vi "HEWH 5 Second After Draw.vi"(6 "Seconds to Remove":T2, 7 "Remove from location":T1, 11 "Software Elapsed Time (s) in":dbl[](array[numeric]) format="%#.6f") -> (2 "Time (15 sec After)":dbl, 3 "Software Elapsed Time (s) out":dbl[](array[numeric]), 4 "Time Index":i32)   [LabVIEW 2023]
uses:
  Type Definitions/HEWH Seconds to Remove.ctl
  Type Definitions/HEWH Remove From Location.ctl
panel:
  out "Difference (Debug)":dbl
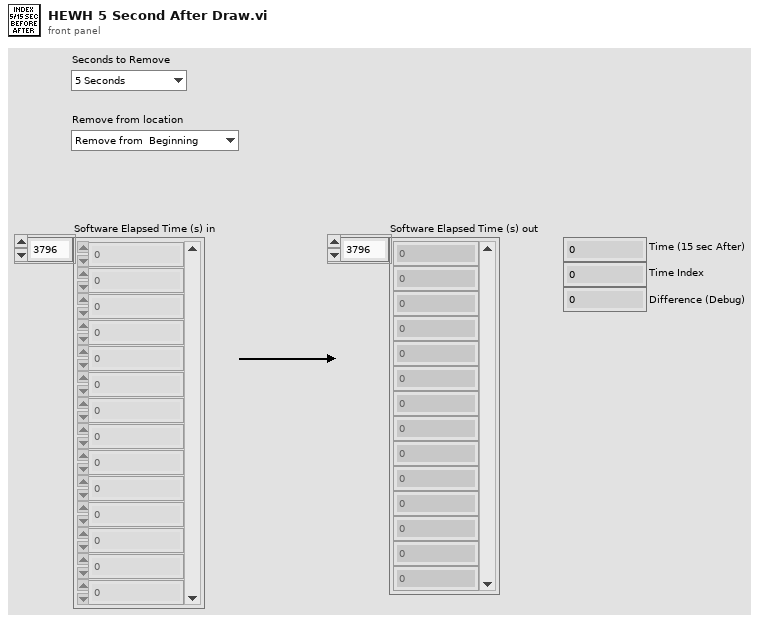
[diagram p1: front panel]
types:
  T1 = typedef "HEWH Remove From Location.ctl" = enum16{"Remove from  Beginning", "Remove from End"}
  T2 = typedef "HEWH Seconds to Remove.ctl" = enum16{"5 Seconds", "15 Seconds"}
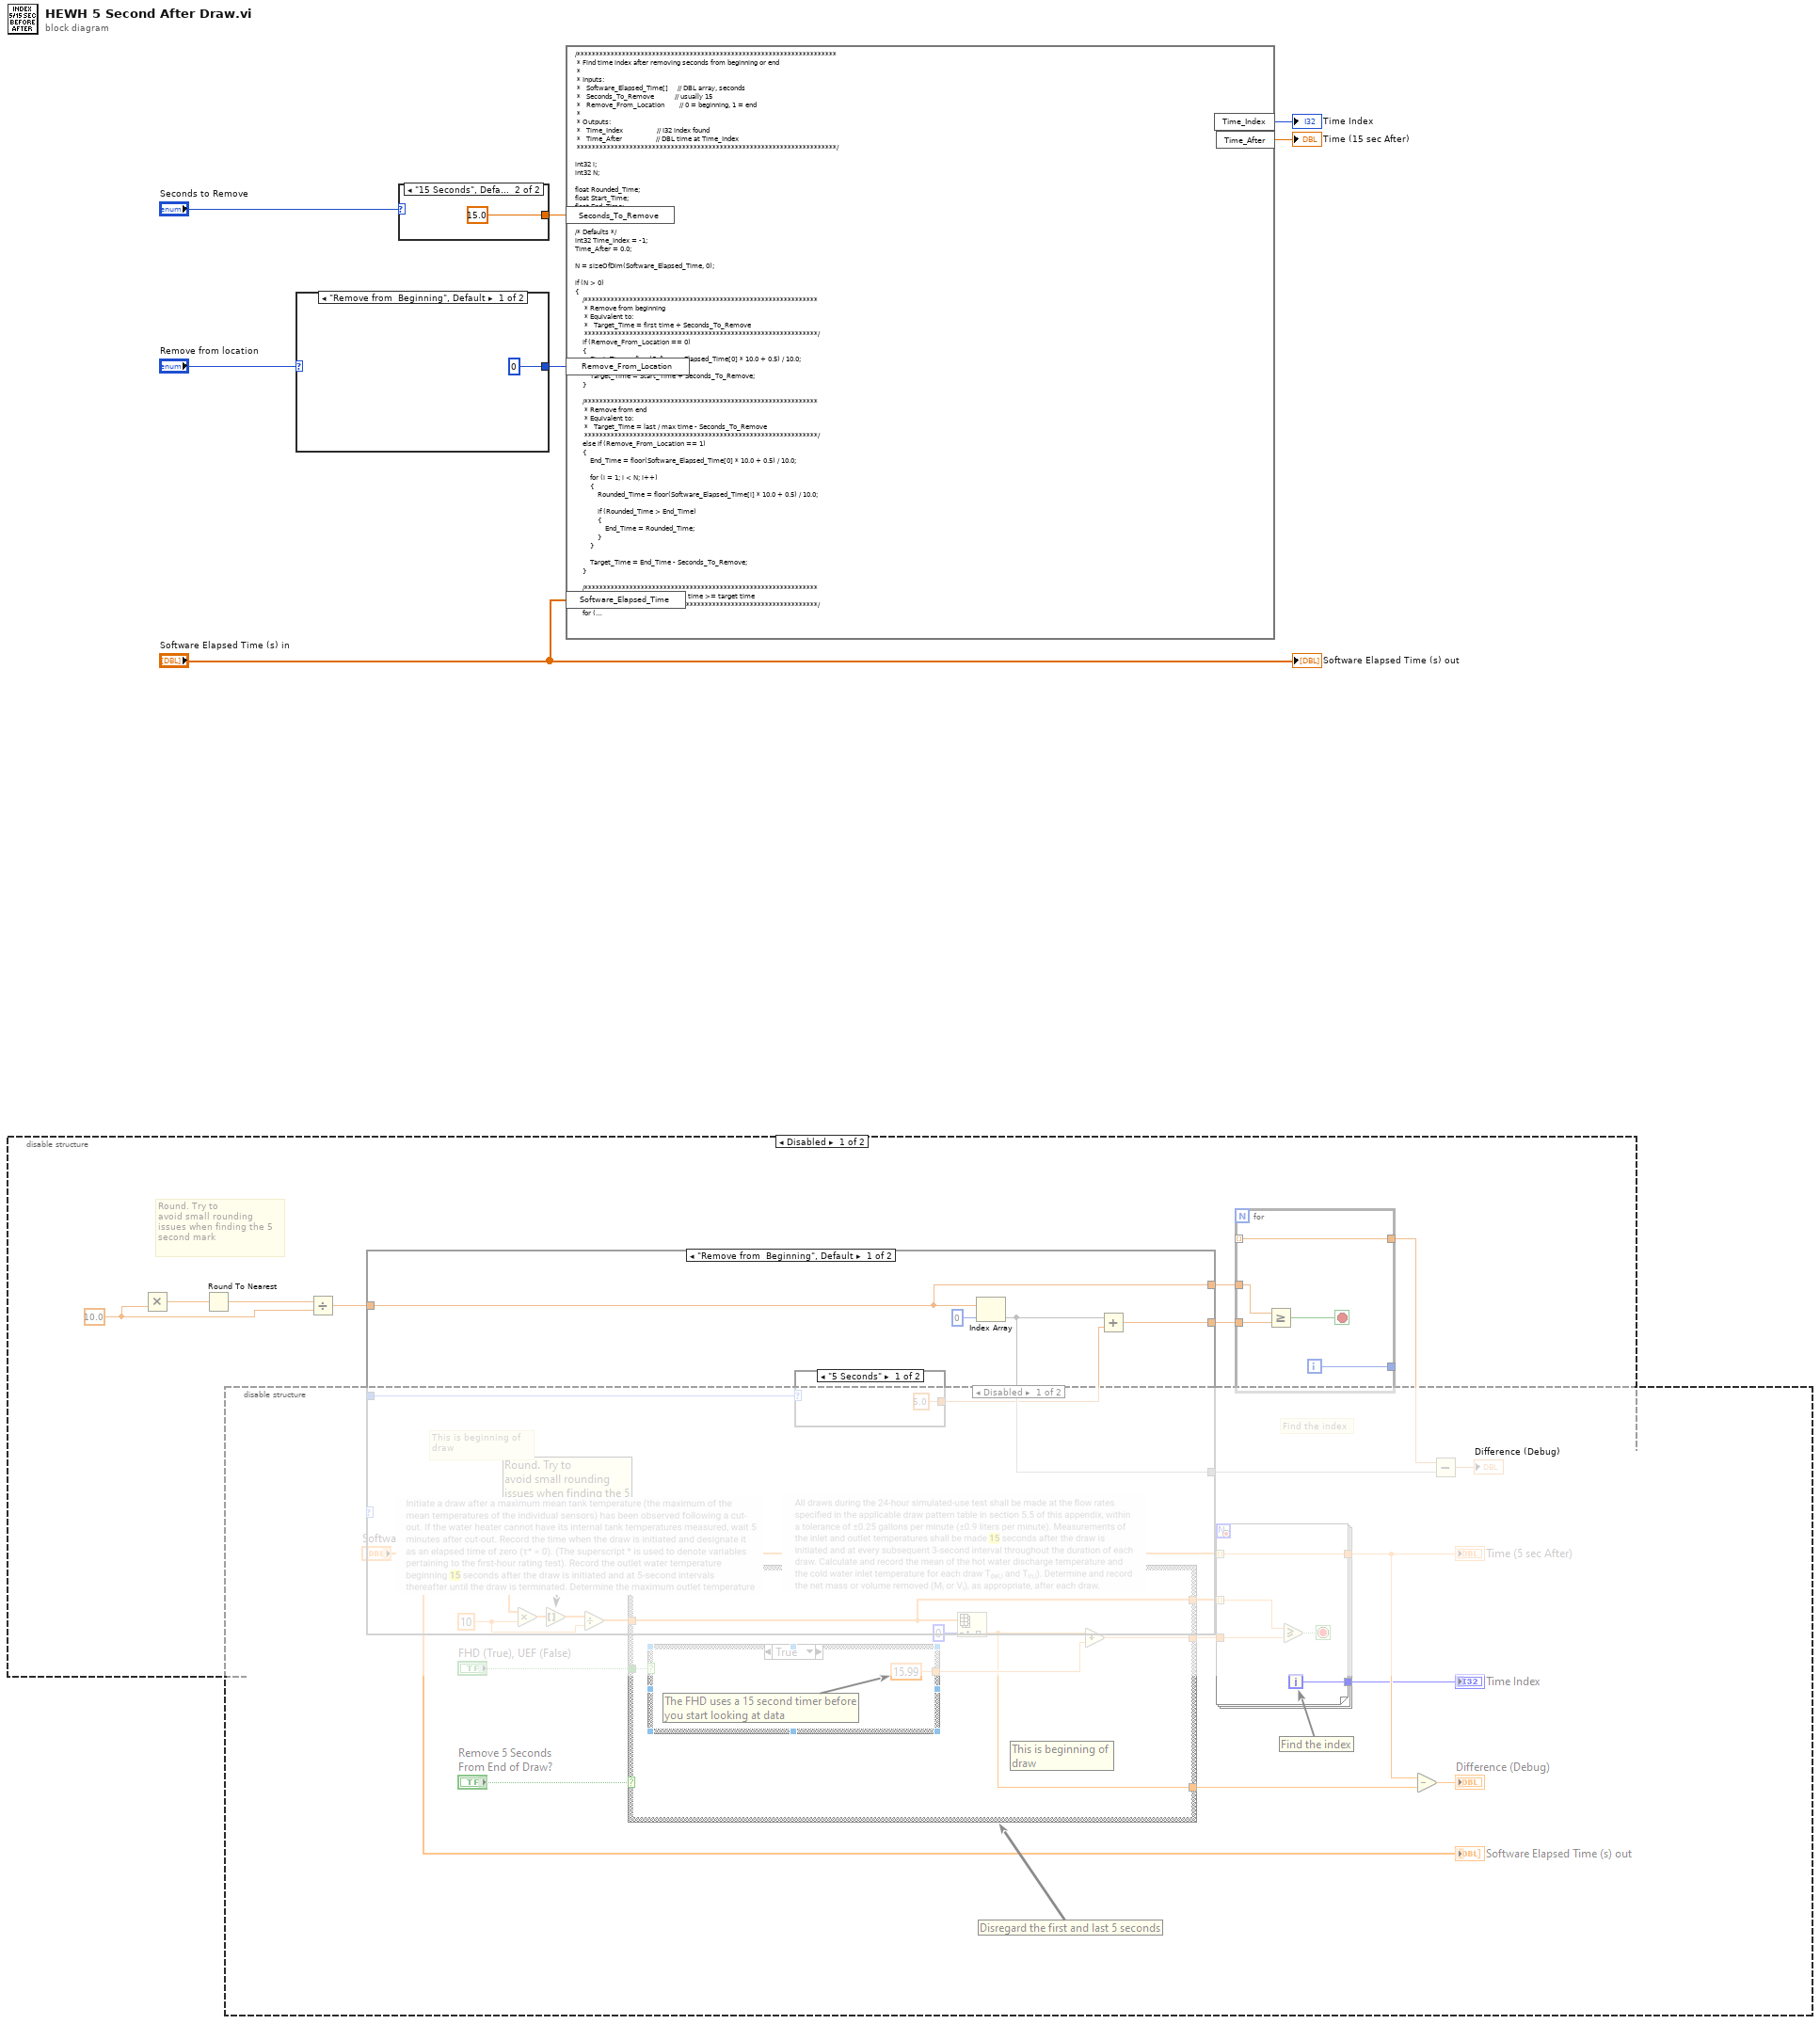
[diagram p0: block diagram]
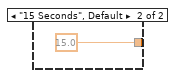
[diagram p2: hidden frame]
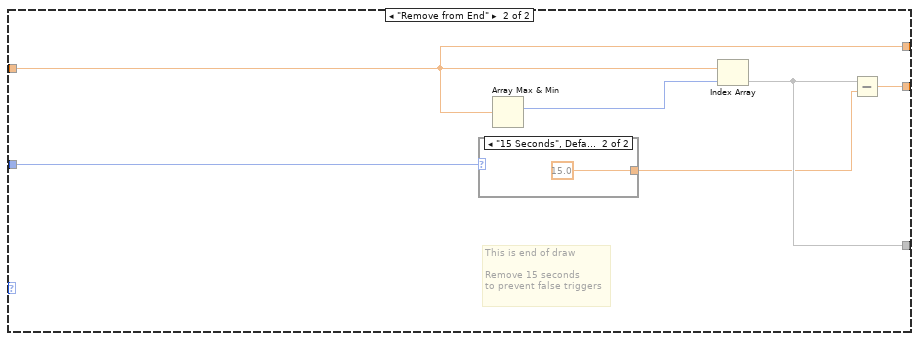
[diagram p3: hidden frame]
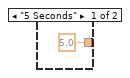
[diagram p4: hidden frame]
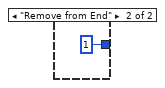
[diagram p6: hidden frame]
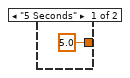
[diagram p7: hidden frame]
diagram:
  n1 = disable-structure shown="Disabled" {
    frame Disabled {
      w16 = 10.0
      # "Find the index"
      # "Round. Try to\navoid small rounding\nissues when finding the 5\nsecond mark"
      n2 = Multiply(y=w16) -> (x*y=w14:dbl)  [unwired: 1 in]
      n3 = Round To Nearest(number=w14) -> (nearest integer value=w15:dbl)
      n4 = Divide(x=w15, y=w16) -> (x/y=w12:dbl)
      n5 = case shown="\"Remove from  Beginning\", Default" {
        selector: _ -> [_ _]
        tunnel: [w22 w30] -> w13
        tunnel: w12 -> [w20 w29]
        tunnel: [w20 w29] -> w11
        tunnel: [w19 w27] -> w9
        tunnel: _ -> [w17 w26]
        frame "Remove from  Beginning", Default {
          # "This is beginning of \ndraw"
          n6 = case shown="\"5 Seconds\"" w17 {
            tunnel: [5.0 ("Ignore Seconds at Beginning") 15.0 ("Ignore Seconds at Beginning")] -> w18
            frame "5 Seconds" {
            }
            frame "15 Seconds", Default {
            }
          }
          n7 = Index Array "Index Array"(array=w20, index=0) -> (element=w19)
          n8 = Add(x=w19, y=w18) -> (x+y=w22:dbl)
        }
        frame "Remove from End" {
          # "This is end of draw\n\nRemove 15 seconds\nto prevent false triggers"
          n9 = case shown="\"15 Seconds\", Default" w26 {
            tunnel: [5.0 ("Ignore Seconds at Beginning") 15.0 ("Ignore Seconds at Beginning")] -> w25
            frame "5 Seconds" {
            }
            frame "15 Seconds", Default {
            }
          }
          n10 = Array Max & Min(array=w29) -> (max index (indices)=w28:i32)  [unwired: 3 out]
          n11 = Index Array(array=w29, index=w28) -> (element=w27)
          n12 = Subtract(x=w27, y=w25) -> (x-y=w30:dbl)
        }
      }
      n13 = for {
        tunnel: w11 -> [w33]
        tunnel: w13 -> [w35]
        tunnel: [w36] -> _
        tunnel: _ -> [w34] mode=indexing
        tunnel: [w34] -> w10
        i -> [w36]
        stop <- w37 stop-if-true
        n14 = Greater Or Equal?(x=w33, y=w35) -> (x >= y?=w37:bool)
      }
      n15 = Subtract(x=w10, y=w9) -> (x-y=→"Difference (Debug)":dbl)
    }
    frame Enabled {
    }
  }
  n16 = disable-structure shown="Disabled" {
    frame Disabled {
    }
    frame Enabled {
    }
  }
  n17 = case shown="\"Remove from  Beginning\", Default" "Remove from location" {
    tunnel: [0 1] -> w4
    frame "Remove from  Beginning", Default {
    }
    frame "Remove from End" {
    }
  }
  n18 = case shown="\"15 Seconds\", Default" "Seconds to Remove" {
    tunnel: [5.0 ("Ignore Seconds at Beginning") 15.0 ("Ignore Seconds at Beginning")] -> w6
    frame "5 Seconds" {
    }
    frame "15 Seconds", Default {
    }
  }
  n19 = formula code="/*********************************************************************\n * Find time index after removing seconds from beginning or end\n *\n * Inputs:\n *   Software_Elapsed_Time[]     // DBL array, seconds\n *   Seconds_To_Remove           // usually 15\n *   Remove_From_Location        // 0 = beginning, 1 = end\n *\n * Outputs:\n *   Time_Index                  // I32 index found\n *   Time_After                  // DBL time at Time_Index\n *********************************************************************/\n\nint32 i;\nint32 N;\n\nfloat Rounded_Time;\nfloat Start_Time;\nfloat End_Time;\nfloat Target_Time;\n\n/* Defaults */\nint32 Time_Index = -1;\nTime_After = 0.0;\n\nN = sizeOfDim(Software_Elapsed_Time, 0);\n\nif (N > 0)\n{\n    /**************************************************************\n     * Remove from beginning\n     * Equivalent to:\n     *   Target_Time = first time + Seconds_To_Remove\n     **************************************************************/\n    if (Remove_From_Location == 0)\n    {\n        Start_Time = floor(Software_Elapsed_Time[0] * 10.0 + 0.5) / 10.0;\n\n        Target_Time = Start_Time + Seconds_To_Remove;\n    }\n\n    /**************************************************************\n     * Remove from end\n     * Equivalent to:\n     *   Target_Time = last / max time - Seconds_To_Remove\n     **************************************************************/\n    else if (Remove_From_Location == 1)\n    {\n        End_Time = floor(Software_Elapsed_Time[0] * 10.0 + 0.5) / 10.0;\n\n        for (i = 1; i < N; i++)\n        {\n            Rounded_Time = floor(Software_Elapsed_Time[i] * 10.0 + 0.5) / 10.0;\n\n            if (Rounded_Time > End_Time)\n            {\n                End_Time = Rounded_Time;\n            }\n        }\n\n        Target_Time = End_Time - Seconds_To_Remove;\n    }\n\n    /**************************************************************\n     * Find first index where rounded time >= target time\n     **************************************************************/\n    for (i = 0; i < N; i++)\n    {\n        Rounded_Time = floor(Software_Elapsed_Time[i] * 10.0 + 0.5) / 10.0;\n\n        if (Rounded_Time >= Target_Time)\n        {\n            Time_Index = i;             // Index in Array where the updated time is located\n            Time_After = Software_Elapsed_Time[i];      //Timestamp in the array\n            break;\n        }\n    }\n}"("Software_Elapsed_Time"="Software Elapsed Time (s) in", "Seconds_To_Remove"=w6, "Remove_From_Location"=w4) -> ("Time_Index"=→"Time Index":i32, "Time_After"=→"Time (15 sec After)":dbl)
  "Software Elapsed Time (s) out" <- "Software Elapsed Time (s) in"
